vi "Right Pre-Buffer Motion Profile Points.vi"(0 "Motor Name":string="Right Drive Master", 5 "Time Conversion Factor":dbl=60.0, 7 "Linear Conversion Factor":dbl=0.32, 9 "Motion Profile Array":dbl[][](array[numeric])=[[0.0, 0.0, 40.0], [-0.08337467825520513, -0.003334987130208205, 40.0], [-0.1390677130201192, -0.008897695651012973, 40.0], [-0.19492455584623336, -0.016694677884862306, 40.0], [-0.2510086591219356, -0.026735024249739732, 40.0], [-0.3073815431496359, -0.039030285975725165, 40.0], [-0.36410243377493184, -0.053594383326722436, 40.0], [-0.42122802815659, -0.07044350445298604, 40.0], [-0.47881240235271993, -0.08959600054709484, 40.0], [-0.5369070673475009, -0.11107228324099487, 40.0], [-0.5955611698912707, -0.1348947300366457, 40.0], [-0.6548218328107405, -0.16108760334907532, 40.0], [-0.7147346113925204, -0.18967698780477613, 40.0], [-0.775344042265126, -0.22069074949538117, 40.0], [-0.8366942543017376, -0.2541585196674507, 40.0], [-0.8988295856916605, -0.2901117030951171, 40.0], [-0.9617951702196142, -0.32858350990390167, 40.0], [-1.0256374015932155, -0.3696090059676303, 40.0], [-1.0904042124755176, -0.413225174466651, 40.0], [-1.1561450345639754, -0.45947097584921004, 40.0], [-1.2229103243391493, -0.508387388822776, 40.0], [-1.2907504489525337, -0.5600174067808774, 40.0], [-1.3597137329803768, -0.6144059561000925, 40.0], [-1.4298433660158398, -0.6715996907407261, 40.0], [-1.501172859832982, -0.7316466051340454, 40.0], [-1.5737196615960474, -0.7945953915978874, 40.0], [-1.6474765630791668, -0.8604944541210541, 40.0], [-1.6909710705266117, -0.9281332969421185, 40.0], [-1.7031955251497082, -0.9962611179481069, 40.0], [-1.7150119402262987, -1.0648615955571588, 40.0], [-1.7262977209957413, -1.1339135043969883, 40.0], [-1.7369143308988308, -1.2033900776329416, 40.0], [-1.7467113222808839, -1.273258530524177, 40.0], [-1.755531834150173, -1.343479803890184, 40.0], [-1.7632194572891051, -1.4140085821817483, 40.0], [-1.769626143271444, -1.4847936279126062, 40.0], [-1.7746206263806816, -1.5557784529678333, 40.0], [-1.778096642045044, -1.6269023186496352, 40.0], [-1.7799801240156299, -1.6981015236102603, 40.0], [-1.7802345886945108, -1.7693109071580408, 40.0], [-1.7788640712878734, -1.8404654700095557, 40.0], [-1.7759132564597238, -1.9115020002679446, 40.0], [-1.771464795537586, -1.982360592089448, 40.0], [-1.7656341524297208, -2.0529859581866368, 40.0], [-1.7585626046542875, -2.1233284623728084, 40.0], [-1.750409190578208, -2.1933448299959366, 40.0], [-1.7413424288334123, -2.262998527149273, 40.0], [-1.7315325353508826, -2.3322598285633083, 40.0], [-1.721144694297844, -2.4011056163352222, 40.0], [-1.710333716296967, -2.4695189649871008, 40.0], [-1.6992402078376685, -2.5374885733006076, 40.0], [-1.6879882035591995, -2.6050081014429756, 40.0], [-1.6766840913772603, -2.672075465098066, 40.0], [-1.665416586872102, -2.73869212857295, 40.0], [-1.6542574979409297, -2.804862428490587, 40.0], [-1.6432630320349335, -2.8705929497719844, 40.0], [-1.6324754210372434, -2.935891966613474, 40.0], [-1.6216549941551943, -3.000758166379682, 40.0], [-1.5813433806965307, -3.064011901607543, 40.0], [-1.5125299404742203, -3.1245130992265118, 40.0], [-1.4449840595853023, -3.1823124616099236, 40.0], [-1.3786130653019146, -3.2374569842220002, 40.0], [-1.3133273687982692, -3.289990078973931, 40.0], [-1.2490420078517022, -3.339951759287999, 40.0], [-1.1856773931728082, -3.3873788550149113, 40.0], [-1.1231595273040005, -3.432305236107071, 40.0], [-1.0614198898664526, -3.4747620317017294, 40.0], [-1.0003951209320594, -3.514777836539012, 40.0], [-0.9400265942226687, -3.5523789003079185, 40.0], [-0.8802599438458972, -3.5875892980617543, 40.0], [-0.8210445827862528, -3.6204310813732046, 40.0], [-0.7623332381956167, -3.650924410901029, 40.0], [-0.7040815197821284, -3.679087671692314, 40.0], [-0.6462475265223379, -3.7049375727532077, 40.0], [-0.5887914948263642, -3.7284892325462624, 40.0], [-0.53167548859271, -3.7497562520899708, 40.0], [-0.4748631261184702, -3.7687507771347097, 40.0], [-0.41831934235020946, -3.785483550828718, 40.0], [-0.3620101811034208, -3.799963958072855, 40.0], [-0.30590261277775055, -3.812200062583965, 40.0], [-0.24996437345339706, -3.8221986375221007, 40.0], [-0.19416382134438517, -3.829965190375876, 40.0], [-0.13846980682687757, -3.835503982648951, 40.0], [-0.0828515529687327, -3.8388180447677005, 40.0], [-0.02752878065815769, -3.839919195994027, 40.0], [0.0, -3.839919195994027, 40.0]], 11 "PIDF Profile Slot Select":u8, 12 "Clear Buffer":bool=TRUE) -> (4 "Ready to Execute":bool)   [LabVIEW 2016]
uses:
  <vilib>/Rock Robotics/WPI/ThirdParty/CanMotor/TalonSRX/WPI_CANTalonSRX_APIControlMode.ctl
  <vilib>/Rock Robotics/WPI/ThirdParty/CanMotor/TalonSRX/WPI_CANTalonSRX_GlobalOps.ctl
  <vilib>/Rock Robotics/WPI/ThirdParty/CanMotor/TalonSRX/WPI_CANTalonSRX_MotionProfileTrajectoryPt.ctl
  Global Variables/MotionProfile.vi
panel:
  out "Initialize Loop Index":i32=86
  out "Initialize Is Last":bool=TRUE
  out "Initialize Mot Prof Count":i32=85
  out "Initialize Mot Prof Buffer Is Full":bool
  out "Total Points in File":i32=86
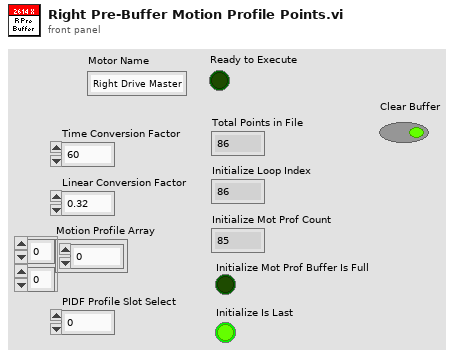
[diagram p1: front panel]
types:
  T1 = typedef "WPI_CANTalonSRX_GlobalOps.ctl" = enum16{"Read For Send", "Write After Receive General", "Write After Receive Feedback", "Write After Receive Encoder", "Write After Receive Ain", "Write Error", "Get All", "Set Output", "Set Mode", "Set Master ID", "Set Brake Mode", "Set Reverse Feedback Sensor", "Set Reverse Closed Loop Output", "Set Override Limits", "Set Forward Limit Enabled", "Set Reverse Limit Enabled", "Set Feedback Select", "Set Profile Select", "Set Throttle Ramp Rate", "Disable", "Set Enc Codes Per Rev", "Set Num Pot Turns", "Set Control Frame Rate", "Enable Legacy Control", "Write After Receive Pulse Width", "Set Enable Frame Rate", "Write After Receive Motion Profile", "Set Motion Profile Flow Control", "Set Motion Profile Control Frame Rate", "Set Current Limit Enable", "Set Usage Frame"}
  T2 = typedef "WPI_CANTalonSRX_APIControlMode.ctl" = enum8{"Percent VBus", "Speed", "Position", "Slave", "Unchanged / Invalid", "Voltage Compensation", "Current", "Motion Profile", "Motion Magic"}
  T3 = typedef "WPI_MotorControlDeviceRef.ctl" = cluster{"DeviceStatus":errorcluster, "Type":T4, "PWM":cluster{"PWM Channel":T5, "DeadBand":T6}, "CAN":cluster{"Device Number":u8, "SetOutput VI Ref":variant, "GetOutput VI Ref":variant, "Enable VI Ref":variant, "Disable VI Ref":variant, "Data":variant}, "Invert":bool}
  T4 = typedef "WPI_MotorControlType.ctl" = enum16{"PWM", "CAN"}
  T5 = typedef "FPGA_DIOPWMChannel.ctl" = enum8{"PWM 0", "PWM 1", "PWM 2", "PWM 3", "PWM 4", "PWM 5", "PWM 6", "PWM 7", "PWM 8", "PWM 9", "PWM MXP 0", "PWM MXP 1", "PWM MXP 2", "PWM MXP 3", "PWM MXP 4", "PWM MXP 5", "PWM MXP 6", "PWM MXP 7", "PWM MXP 8", "PWM MXP 9", "Invalid"}
  T6 = typedef "WPI_PWMDeadband.ctl" = cluster{"Name":string, "maxPositivePwm":i32, "minPositivePwm":i32, "centerPwm":i32, "maxNegativePwm":i32, "minNegativePwm":i32, "angularRange":u16}
  T7 = typedef "WPI_CANTalonSRX_MotionProfileTrajectoryPt.ctl" = cluster{"Duration Ms":u8, "Velocity":dbl, "Position":dbl, "Profile Slot Select":u8, "Is Last":bool, "Velocity Only":bool, "Zero Position":bool, "Compress Code":u8, "Same Velocity":i32, "Delta Position":i32, "Count":u8}
  T8 = typedef "MotionProfile TypeDef.ctl" = cluster{"Left MP Array":dbl[][], "Left MP Index":dbl, "Semaphore":bool, "Right MP Array":dbl[][], "Right MP Index":dbl}
  T9 = typedef "WPI_CANTalonSRX_GlobalStatus.ctl" = cluster{"Applied Throttle":dbl, "Module Enabled":bool, "CAN Error":errorcluster, "Closed Loop Error":dbl, "Forward Limit Switch Closed":bool, "Reverse Limit Switch Closed":bool, "Sensor Position":dbl, "Sensor Velocity":dbl, "Current":dbl, "Sticky Fault - Over Temp":bool, "Sticky Fault - Under Voltage":bool, "Sticky Fault - Forward Limit":bool, "Sticky Fault - Reverse Limit":bool, "Sticky Fault - Forward Soft Limit":bool, "Sticky Fault - Reverse Soft Limit":bool, "Brake is Enabled":bool, "Encoder Position":dbl, "Encoder Velocity":dbl, "Encoder Index Count":dbl, "Encoder A Pin State":bool, "Encoder B Pin State":bool, "Encoder Index Pin State":bool, "Analog In":dbl, "Analog In Velocity":dbl, "Temperature (C)":dbl, "Battery Voltage":dbl, "Control 5 Is Supported":bool, "Current Profile Slot Select":dbl, "Pos Div 8":bool, "Vel Div 4":bool, "Pulse Width Position":i32, "Pulse Width Velocity":i32, "Pulse Width Rise To Rise (us)":i32, "Pulse Width Rise To Fall (us)":i32, "Mot Prof Active Is Under Run":bool, "Mot Prof Active Has Under Run":bool, "Mot Prof Active Is Last":bool, "Mot Prof Active Velocity Only":bool, "Mot Prof Active Is Valid":bool, "Mot Prof Buffer Is Full":bool, "Mot Prof Active Profile Slot Select":i32, "Mot Prof NextID":i32, "Mot Prof Count":i32, "Mot Prof Active Velocity":dbl, "Mot Prof Active Position":dbl, "Mot Prof Output Enable":i32, "UsageFrame":u32}
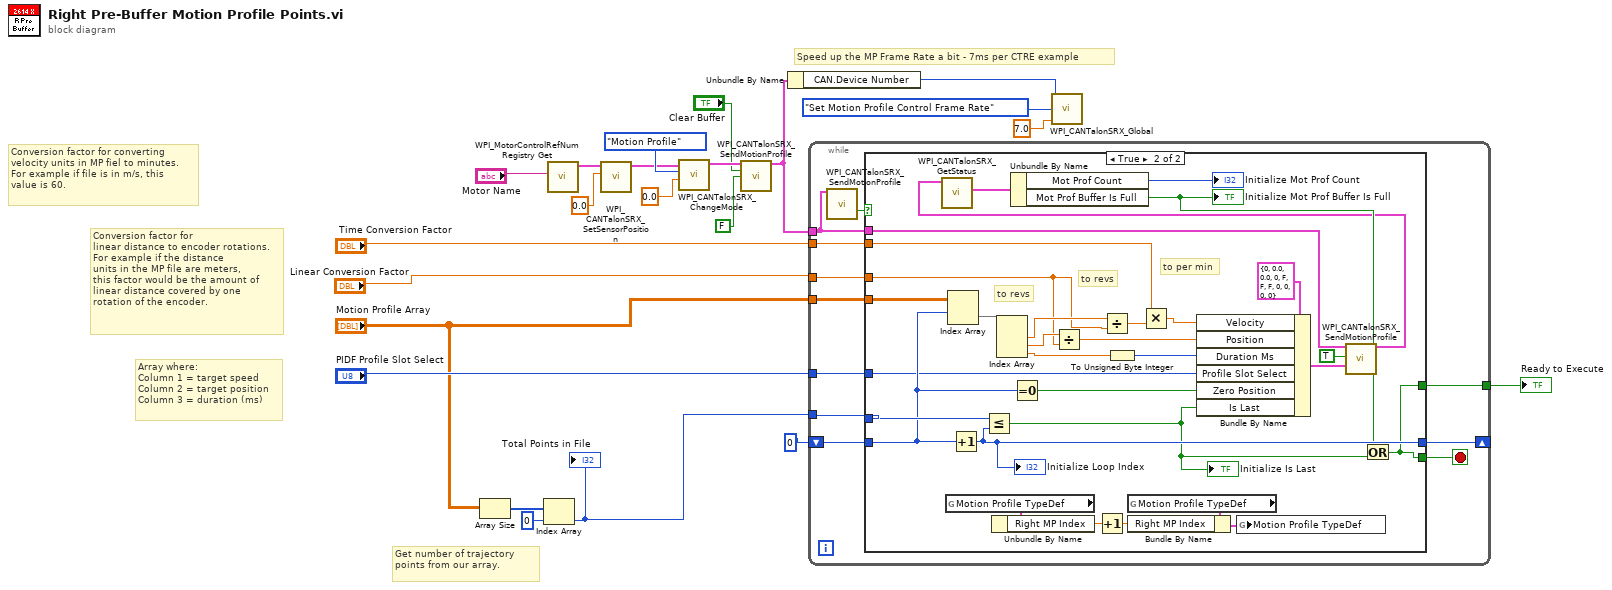
[diagram p0: block diagram]
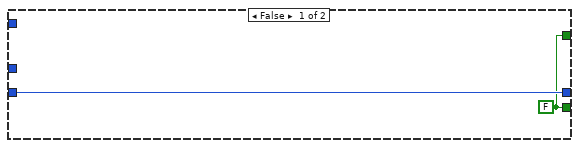
[diagram p2: hidden frame]
diagram:
  # "Array where:\nColumn 1 = target speed\nColumn 2 = target position\nColumn 3 = duration (ms)"
  # "Conversion factor for converting \nvelocity units in MP fiel to minutes.\nFor example if file is in m/s, this\nvalue is 60."
  # "Conversion factor for\nlinear distance to encoder rotations.\nFor example if the distance\nunits in the MP file are meters,\nthis factor would be the amount of\nlinear distance covered by one\nrotation of the encoder."
  # "Speed up the MP Frame Rate a bit - 7ms per CTRE example"
  # "Get number of trajectory points from our array."
  n1 = Array Size(array="Motion Profile Array") -> (size(s)=w17:i32[])
  n2 = Index Array(array=w17, index=0) -> (element=w13:i32)
  "Total Points in File" <- w13
  n3 = call <vilib>:"WPI_MotorControlRefNum Registry Get.vi"("refnum name"="Motor Name") -> ("MotorControlDevRef"=w22:T3)  [unwired: 9 in, 1 out]
  n4 = call <vilib>:"WPI_CANTalonSRX_SetSensorPosition.vi"("New Sensor Position"=0.0, "CAN Talon SRX Ref"=w22) -> ("CAN Talon SRX Ref"=w18:T3)  [unwired: 8 in, 1 out]
  n5 = call <vilib>:"WPI_CANTalonSRX_ChangeMode.vi"("Output"=0.0, "Control Mode"=WPI_CANTalonSRX_APIControlMode."Motion Profile", "CAN Talon SRX Ref"=w18) -> ("CAN Talon SRX Ref"=w15:T3)  [unwired: 7 in, 1 out]
  n6 = call <vilib>:"WPI_CANTalonSRX_SendMotionProfile.vi"("CAN Talon SRX Ref"=w15, "Clear"="Clear Buffer", "Push"=FALSE) -> ("CAN Talon SRX Ref Out"=w11:T3)  [unwired: 9 in, 3 out]
  n7 = Unbundle By Name(w11) -> ("CAN.Device Number"=w10:u8)
  n8 = while {
    tunnel: w11 -> [w26]
    shift-right: [w32] -> _
    shift-left: 0 -> [w30]
    tunnel: w13 -> [w33]
    tunnel: "Motion Profile Array" -> [w31]
    tunnel: "Linear Conversion Factor" -> [w29]
    tunnel: "Time Conversion Factor" -> [w28]
    tunnel: "PIDF Profile Slot Select" -> [w27]
    tunnel: [w23] -> w3
    stop <- w24 stop-if-true
    n9 = call <vilib>:"WPI_CANTalonSRX_SendMotionProfile.vi"("CAN Talon SRX Ref"=w26) -> ("Ready For Next"=w25:bool)  [unwired: 11 in, 3 out]
    n10 = case shown="True" w25 {
      tunnel: w33 -> [_ w66]
      tunnel: [w35 w65] -> w32
      tunnel: w31 -> [_ w59]
      tunnel: w30 -> [w35 w58]
      tunnel: w29 -> [_ w55]
      tunnel: w28 -> [_ w48]
      tunnel: w27 -> [_ w47]
      tunnel: w26 -> [_ w45]
      tunnel: [w34 w43] -> w24
      tunnel: [w34 w43] -> w23
      frame False {
        w34 = FALSE
      }
      frame True {
        # "to per min"
        # "to revs"
        # "to revs"
        n11 = global read "MotionProfile.vi" "Motion Profile TypeDef"() -> (w36:T8)
        n12 = Index Array(array=w59, index (row)=w58) -> (element=w60:dbl[])  [unwired: 1 in]
        n13 = Increment(x=w58) -> (x+1=w65:i32)
        "Initialize Loop Index" <- w65
        n14 = Less Or Equal?(x=w66, y=w65) -> (x <= y?=w41:bool)
        "Initialize Is Last" <- w41
        n15 = Unbundle By Name(w36) -> ("Right MP Index"=w39:dbl)
        n16 = Index Array(array=w60) -> (element #1=w57:dbl, element #2=w56:dbl, element #3=w50:dbl)  [unwired: 3 in]
        n17 = Equal To 0?(x=w58) -> (x = 0?=w62:bool)
        n18 = Divide(x=w56, y=w55) -> (x/y=w52:dbl)
        n19 = Increment(x=w39) -> (x+1=w40:dbl)
        n20 = Divide(x=w57, y=w55) -> (x/y=w54:dbl)
        n21 = To Unsigned Byte Integer(number=w50) -> (unsigned 8bit integer=w49:u8)
        n22 = global read "MotionProfile.vi" "Motion Profile TypeDef"() -> (w37:T8)
        n23 = Bundle By Name(cluster=w37, "Right MP Index"=w40) -> (w38:T8)
        n24 = Multiply(x=w48, y=w54) -> (x*y=w53:dbl)
        n25 = Bundle By Name(cluster=T7 {"Duration Ms"=0, "Velocity"=0.0, "Position"=0.0, "Profile Slot Select"=0, "Is Last"=FALSE, "Velocity Only"=FALSE, "Zero Position"=FALSE, "Compress Code"=0, "Same Velocity"=0, "Delta Position"=0, "Count"=0} ("New Point"), "Velocity"=w53, "Position"=w52, "Duration Ms"=w49, "Profile Slot Select"=w47, "Zero Position"=w62, "Is Last"=w41) -> (w63:T7)
        n26 = global write "MotionProfile.vi" "Motion Profile TypeDef"(w38) -> ()
        n27 = call <vilib>:"WPI_CANTalonSRX_SendMotionProfile.vi"("CAN Talon SRX Ref"=w45, "Push"=TRUE, "New Point"=w63) -> ("CAN Talon SRX Ref Out"=w42:T3)  [unwired: 9 in, 3 out]
        n28 = call <vilib>:"WPI_CANTalonSRX_GetStatus.vi"("CAN Talon SRX Ref"=w42) -> ("Talon SRX Status"=w51:T9)  [unwired: 8 in, 2 out]
        n29 = Unbundle By Name(w51) -> ("Mot Prof Count"=→"Initialize Mot Prof Count":i32, "Mot Prof Buffer Is Full"=w44:bool)
        "Initialize Mot Prof Buffer Is Full" <- w44
        n30 = Or(x=w44, y=w41) -> (x .or. y?=w43:bool)
      }
    }
  }
  "Ready to Execute" <- w3
  n31 = call <vilib>:"WPI_CANTalonSRX_Global.vi"("Set Number"=7.0, "Operation"=WPI_CANTalonSRX_GlobalOps."Set Motion Profile Control Frame Rate", "Device ID (0)"=w10) -> ()  [unwired: 6 in, 3 out]
